vi "LP Check Motors limits.vi"(10 "RollPos":dbl, 11 "PitchPos":dbl) -> (2 "RollLimit+":bool, 3 "PitchLimit+":bool)   [LabVIEW 2015]
uses:
  Stream/LP Globals.vi
panel:
  out "PitchLimit-":bool
  out "RollLimit-":bool
  out "Quarter":u8
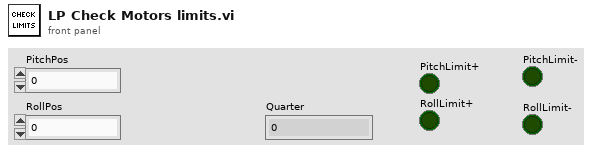
[diagram p1: front panel]
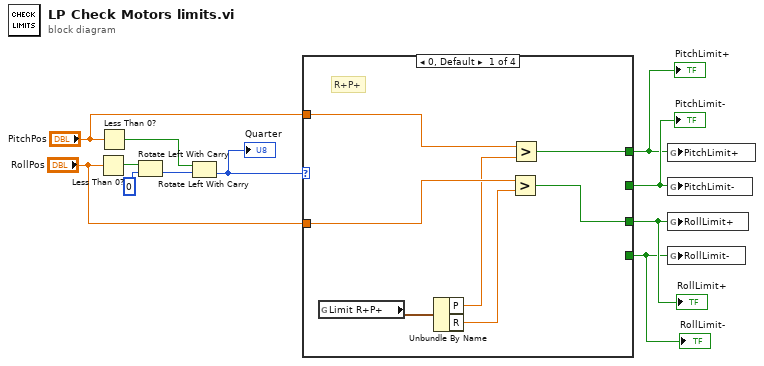
[diagram p0: block diagram]
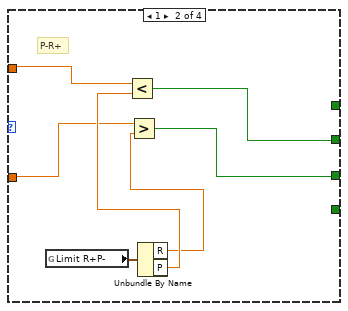
[diagram p2: hidden frame]
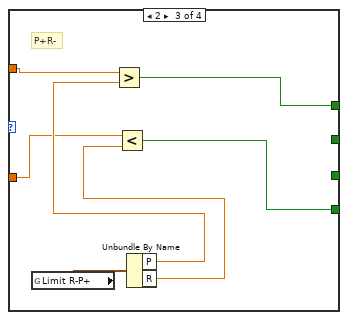
[diagram p3: hidden frame]
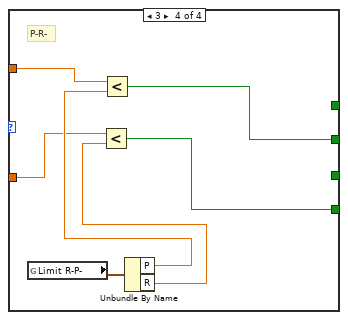
[diagram p4: hidden frame]
diagram:
  n1 = Less Than 0?(x="RollPos") -> (x < 0?=w9:bool)
  n2 = Less Than 0?(x="PitchPos") -> (x < 0?=w8:bool)
  n3 = Rotate Left With Carry(2:u8 0, 3:w9) -> (0:w10:u8)  [unwired: 1 out]
  n4 = Rotate Left With Carry(2:w10, 3:w8) -> (0:w7:u8)  [unwired: 1 out]
  "Quarter" <- w7
  n5 = case shown="0, Default" w7 {
    tunnel: "PitchPos" -> [w17 w24 w31 w39]
    tunnel: "RollPos" -> [w16 w22 w29 w36]
    tunnel: [w13 _ w27 _] -> w3
    tunnel: [_ w20 _ w34] -> w4
    tunnel: [_ _ w26 w33] -> w1
    tunnel: [w12 w19 _ _] -> w2
    frame 0, Default {
      # "R+P+"
      n6 = global read "LP Globals.vi" "Limit R+P+"() -> (w18:cluster{"R":dbl, "P":dbl})
      n7 = Unbundle By Name(w18) -> ("P"=w15:dbl, "R"=w14:dbl)
      n8 = Greater?(x=w16, y=w14) -> (0:w12:bool)
      n9 = Greater?(x=w17, y=w15) -> (0:w13:bool)
    }
    frame 1 {
      # "P-R+"
      n10 = global read "LP Globals.vi" "Limit R+P-"() -> (w25:cluster{"R":dbl, "P":dbl})
      n11 = Unbundle By Name(w25) -> ("R"=w21:dbl, "P"=w23:dbl)
      n12 = Less?(x=w24, y=w23) -> (x < y?=w20:bool)
      n13 = Greater?(x=w22, y=w21) -> (0:w19:bool)
    }
    frame 2 {
      # "P+R-"
      n14 = global read "LP Globals.vi" "Limit R-P+"() -> (w32:cluster{"R":dbl, "P":dbl})
      n15 = Unbundle By Name(w32) -> ("P"=w30:dbl, "R"=w28:dbl)
      n16 = Greater?(x=w31, y=w30) -> (0:w27:bool)
      n17 = Less?(x=w29, y=w28) -> (x < y?=w26:bool)
    }
    frame 3 {
      # "P-R-"
      n18 = global read "LP Globals.vi" "Limit R-P-"() -> (w38:cluster{"R":dbl, "P":dbl})
      n19 = Unbundle By Name(w38) -> ("P"=w37:dbl, "R"=w35:dbl)
      n20 = Less?(x=w36, y=w35) -> (x < y?=w33:bool)
      n21 = Less?(x=w39, y=w37) -> (x < y?=w34:bool)
    }
  }
  "PitchLimit+" <- w3
  "RollLimit+" <- w2
  "RollLimit-" <- w1
  "PitchLimit-" <- w4
  n22 = global write "LP Globals.vi" "PitchLimit+"(w3) -> ()
  n23 = global write "LP Globals.vi" "PitchLimit-"(w4) -> ()
  n24 = global write "LP Globals.vi" "RollLimit+"(w2) -> ()
  n25 = global write "LP Globals.vi" "RollLimit-"(w1) -> ()
